vi "Release.vi"(8 "error in (no error)":errorcluster, 9 "force destroy? (F)":bool, 11 "Queue in":refnum<class "Queue.lvclass">) -> (0 "error out":errorcluster, 2 "Remaining element":refnum<class "Data.lvclass">[](array[class]), 3 "Queue name":string)   [LabVIEW 2020, in "Data.lvlib" / "Queue.lvclass"]
doc: "Release the queue."
uses:
  Queue.lvclass
  Data.lvclass
  Queue.lvclass/Queue.ctl
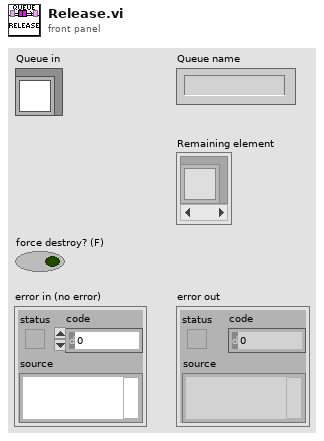
[diagram p1: front panel]
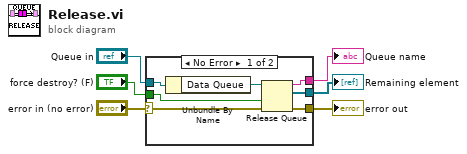
[diagram p0: block diagram]
diagram:
  n1 = case shown="No Error" "error in (no error)" {
    selector: "error in (no error)" -> [w12 w14]
    tunnel: [w11 w14] -> w5
    tunnel: [w8 _] -> w3
    tunnel: "Queue in" -> [w13 _]
    tunnel: [w10 _] -> w2
    tunnel: "force destroy? (F)" -> [w7 _]
    frame No Error {
      n2 = Unbundle By Name(w13) -> ("Data Queue"=w9:refnum<queue>)
      n3 = Release Queue(queue=w9, force destroy? (F)=w7, error in (no error)=w12) -> (queue name=w8:string, remaining elements=w10:refnum<class "Data.lvclass">[], error out=w11:errorcluster)
    }
    frame Error {
    }
  }
  "error out" <- w5
  "Queue name" <- w3
  "Remaining element" <- w2
